vi "simon says.vi"() -> ()   [LabVIEW 2015]
uses:
  <vilib>/rvi/interface/nirviOpenFPGA/nirviOpenFPGA.xnode
  FPGA Bitfiles/ExamenParcial1PD_FPGATarget_kkk_HW3B5lqQ4pI.lvbitx
  <vilib>/rvi/interface/nirviReadWriteControl/nirviReadWriteControl.xnode
  NiFpgaLv.dll
  <vilib>/Utility/error.llb/Error Cluster From Error Code.vi
  <vilib>/rvi/interface/Simulation/niFpgaSimulationCallBeginRW.vi
  <vilib>/rvi/errors/niLvFpgaAdjustHostInterfaceError.vi
  <vilib>/FPGAPlugInAG/sbRIO-9636/niLvFpga_Open_sbRIO-9636.vi
  <vilib>/rvi/interface/common/dynamic/niFpgaDynamicAddResources.vi
panel:
  out "Press that button!":u32(slide) scale=0.0..1000.0
  out "?":bool
  out "?":bool
  out "?":bool
  out "?":bool
  out "?":bool
  out "?":bool
  out "?":bool
  out "?":bool
  out "j 4":bool
  out "J 3":bool
  out "j 2":bool
  out "j 1":bool
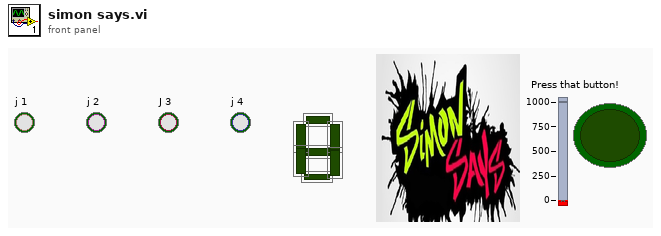
[diagram p1: front panel]
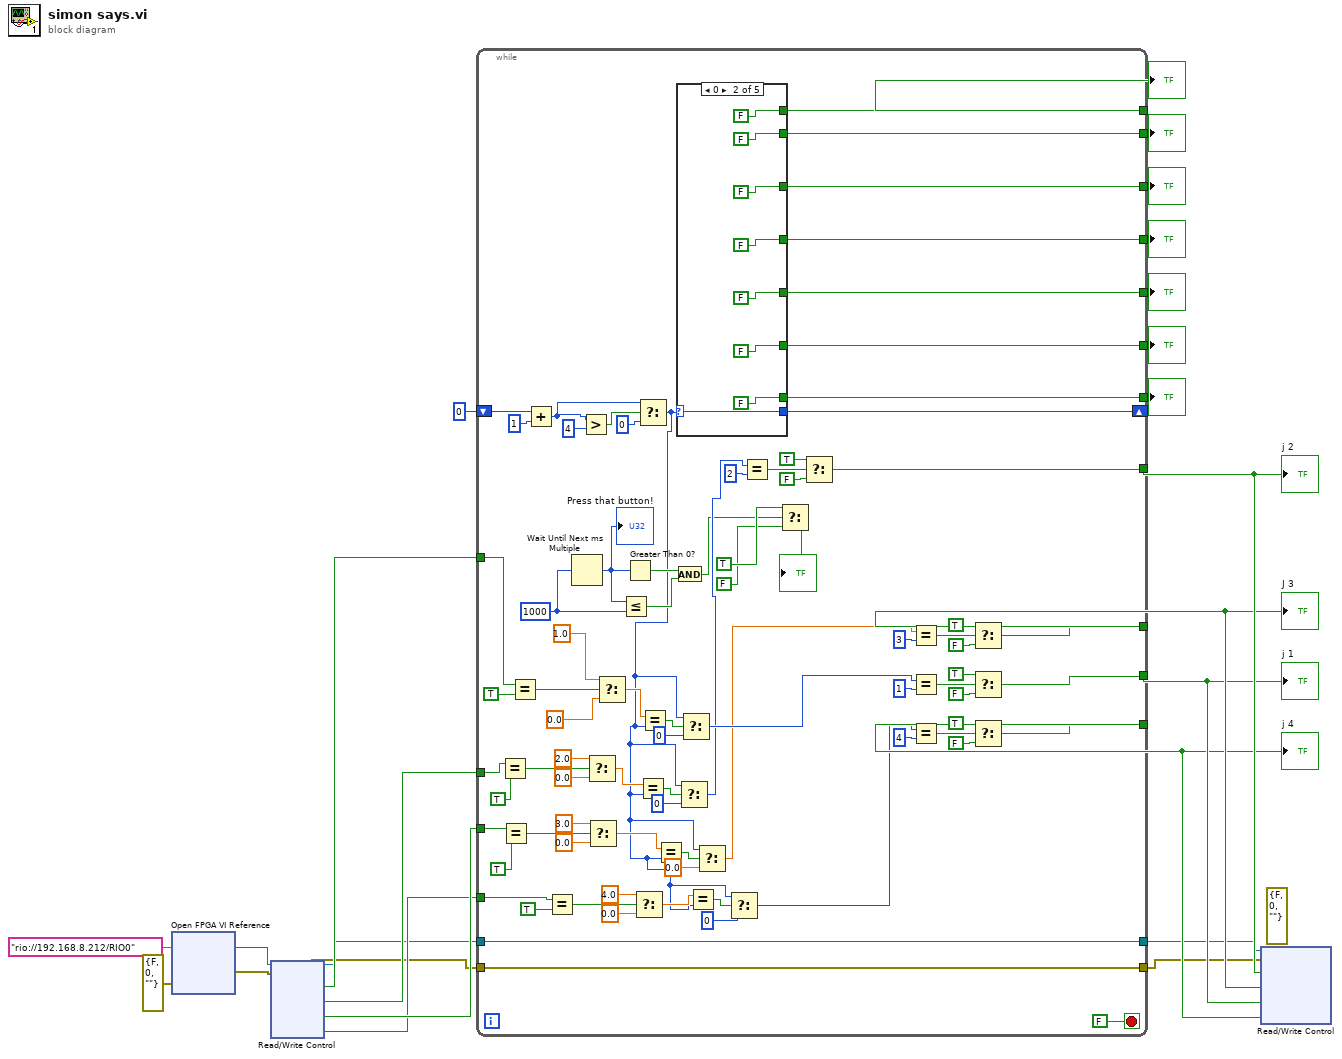
[diagram p0: block diagram]
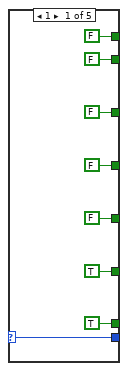
[diagram p2: hidden frame]
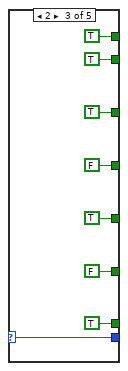
[diagram p3: hidden frame]
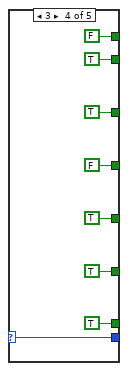
[diagram p4: hidden frame]
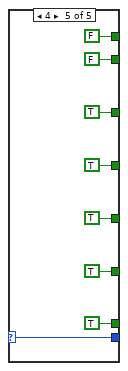
[diagram p5: hidden frame]
diagram:
  (unwired) errorcluster {"status"=FALSE, "code"=0, "source"=""} ("error out")
  n1 = xnode "Open FPGA VI Reference"("error in"=errorcluster {"status"=FALSE, "code"=0, "source"=""}, "resource name"=tag "rio://192.168.8.212/RIO0") -> ("FPGA VI Reference Out"=w16:refnum<k20>, "error out"=w15:errorcluster)
  n2 = xnode "Read/Write Control"("FPGA VI Reference In"=w16, "error in"=w15) -> ("FPGA VI Reference Out"=w4:refnum<k20>, "error out"=w2:errorcluster, "led2"=w14:bool, "led4"=w13:bool, "led1"=w12:bool, "led3"=w11:bool)
  n3 = while {
    shift-right: [w103] -> _
    shift-left: 0 -> [w106]
    tunnel: [w102] -> w23
    tunnel: [w101] -> w22
    tunnel: [w100] -> w21
    tunnel: [w99] -> w20
    tunnel: [w98] -> w19
    tunnel: [w97] -> w18
    tunnel: [w96] -> w17
    tunnel: [w79] -> w6
    tunnel: [w78] -> w8
    tunnel: [w77] -> w7
    tunnel: [w76] -> w5
    tunnel: w14 -> [w65]
    tunnel: w13 -> [w51]
    tunnel: w12 -> [w50]
    tunnel: w11 -> [w47]
    tunnel: w4 -> [w26]
    tunnel: [w26] -> w3
    tunnel: w2 -> [w25]
    tunnel: [w25] -> w1
    stop <- FALSE stop-if-true
    w73 = u32 1000 ("millisecond multiple")
    n4 = Equal?(x=w51, y=TRUE) -> (x = y?=w52:bool)
    n5 = Equal?(x=w50, y=TRUE) -> (x = y?=w55:bool)
    n6 = Equal?(x=w65, y=TRUE) -> (x = y?=w67:bool)
    n7 = Add(x=w106, y=1) -> (x+y=w28:i32)
    n8 = Equal?(x=w47, y=TRUE) -> (x = y?=w59:bool)
    n9 = Wait Until Next ms Multiple(millisecond multiple=w73) -> (millisecond timer value=w74:u32)
    "Press that button!" <- w74
    n10 = Greater?(x=w28, y=4) -> (0:w27:bool)
    n11 = Select(t=2.0, s=w52, f=0.0) -> (s? t:f=w46:dbl)
    n12 = Select(t=3.0, s=w55, f=0.0) -> (s? t:f=w44:dbl)
    n13 = Select(t=1.0, s=w67, f=0.0) -> (s? t:f=w63:dbl)
    n14 = Less Or Equal?(x=w74, y=w73) -> (x <= y?=w72:bool)
    n15 = Greater Than 0?(x=w74) -> (x > 0?=w75:bool)
    n16 = Select(t=4.0, s=w59, f=0.0) -> (s? t:f=w43:dbl)
    n17 = Select(t=w28, s=w27, f=0) -> (s? t:f=w37:i32)
    n18 = Equal?(x=w46, y=w37) -> (x = y?=w45:bool)
    n19 = Equal?(x=w63, y=w37) -> (x = y?=w62:bool)
    n20 = Equal?(x=w44, y=w37) -> (x = y?=w41:bool)
    n21 = And(x=w75, y=w72) -> (x .and. y?=w30:bool)
    n22 = case shown="0" w37 {
      selector: w37 -> [w114 w122 w128 w138 w139]
      tunnel: [w114 w122 w128 w138 w139] -> w103
      tunnel: [TRUE FALSE TRUE TRUE TRUE] -> w102
      tunnel: [TRUE FALSE FALSE TRUE TRUE] -> w101
      tunnel: [FALSE FALSE TRUE TRUE TRUE] -> w100
      tunnel: [FALSE FALSE FALSE FALSE TRUE] -> w99
      tunnel: [FALSE FALSE TRUE TRUE TRUE] -> w98
      tunnel: [FALSE FALSE TRUE TRUE FALSE] -> w97
      tunnel: [FALSE FALSE TRUE FALSE FALSE] -> w96
      frame 1 {
      }
      frame 0 {
      }
      frame 2 {
      }
      frame 3 {
      }
      frame 4 {
      }
    }
    n23 = Select(t=w37, s=w45, f=0) -> (s? t:f=w34:i32)
    n24 = Select(t=w37, s=w62, f=0) -> (s? t:f=w35:i32)
    n25 = Equal?(x=w43, y=w37) -> (x = y?=w42:bool)
    n26 = Select(t=w37, s=w41, f=0.0) -> (s? t:f=w33:dbl)
    n27 = Select(t=w37, s=w42, f=0) -> (s? t:f=w32:i32)
    n28 = Equal?(x=w34, y=2) -> (x = y?=w91:bool)
    n29 = Select(t=TRUE, s=w30, f=FALSE) -> (s? t:f=→"?":bool)
    n30 = Select(t=TRUE, s=w91, f=FALSE) -> (s? t:f=w78:bool)
    n31 = Equal?(x=w33, y=3) -> (x = y?=w83:bool)
    n32 = Equal?(x=w35, y=1) -> (x = y?=w88:bool)
    n33 = Equal?(x=w32, y=4) -> (x = y?=w80:bool)
    n34 = Select(t=TRUE, s=w83, f=FALSE) -> (s? t:f=w77:bool)
    n35 = Select(t=TRUE, s=w88, f=FALSE) -> (s? t:f=w79:bool)
    n36 = Select(t=TRUE, s=w80, f=FALSE) -> (s? t:f=w76:bool)
  }
  "?" <- w19
  "?" <- w21
  "?" <- w23
  "?" <- w18
  "?" <- w22
  "?" <- w20
  "?" <- w17
  "j 1" <- w6
  "j 2" <- w8
  "J 3" <- w7
  "j 4" <- w5
  n37 = xnode "Read/Write Control"("FPGA VI Reference In"=w3, "error in"=w1, "Boolean 4"=w8, "Boolean 3"=w7, "Boolean 3"=w6, "Boolean"=w5) -> ()  [unwired: 2 out]
